vi "YMD.vi"() -> (0 "DD":string, 1 "MM":string, 2 "YYYY":string)   [LabVIEW 2013]
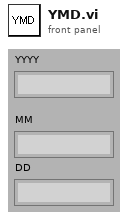
[diagram p1: front panel]
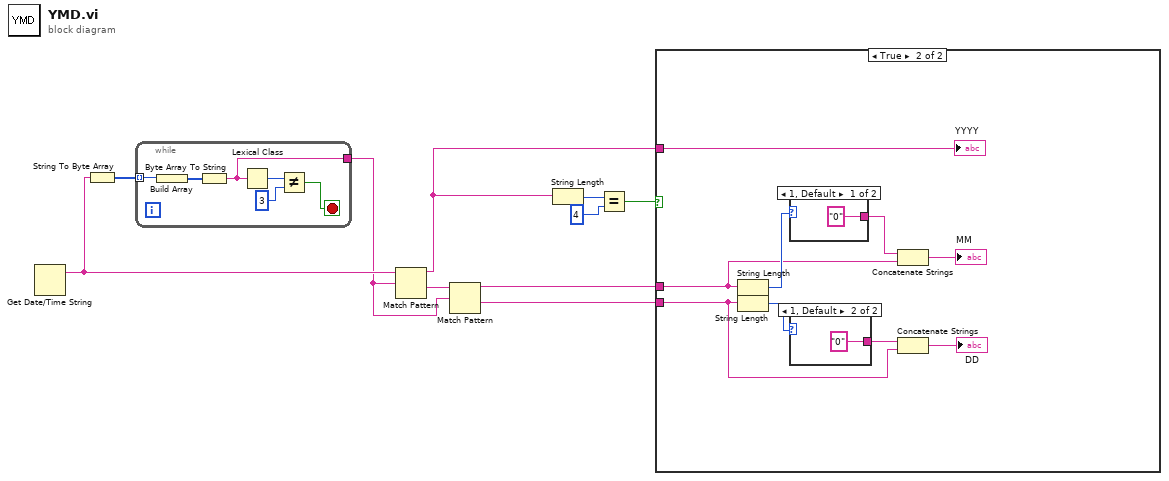
[diagram p0: block diagram]
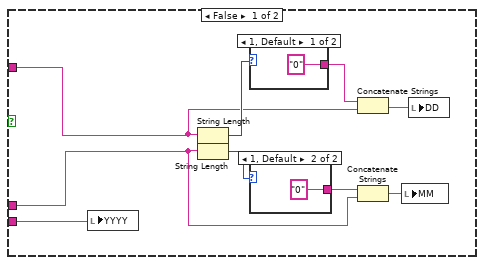
[diagram p2: hidden frame]
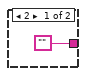
[diagram p3: hidden frame]
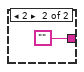
[diagram p4: hidden frame]
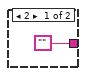
[diagram p5: hidden frame]
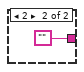
[diagram p6: hidden frame]
diagram:
  n1 = Get Date/Time String() -> (date string=w7:string)  [unwired: 4 out]
  n2 = String To Byte Array(string=w7) -> (unsigned byte array=w6:u8[])
  n3 = while {
    tunnel: w6 -> [w16] mode=indexing
    tunnel: [w11] -> w5
    stop <- w12 stop-if-true
    n4 = Build Array(w16) -> (w15:u8[])
    n5 = Byte Array To String(unsigned byte array=w15) -> (string=w11:string)
    n6 = Lexical Class(1:w11) -> (0:w14:i16)
    n7 = Not Equal?(x=w14, y=3) -> (x != y?=w12:bool)
  }
  n8 = Match Pattern(string=w7, regular expression=w5) -> (before substring=w4:string, after substring=w8:string)  [unwired: 3 out]
  n9 = Match Pattern(string=w8, regular expression=w5) -> (before substring=w9:string, after substring=w10:string)  [unwired: 3 out]
  n10 = String Length(string=w4) -> (length=w3:i32)
  n11 = Equal?(x=w3, y=4) -> (x = y?=w1:bool)
  n12 = case shown="True" w1 {
    tunnel: w10 -> [w19 w35]
    tunnel: w9 -> [w20 w33]
    tunnel: w4 -> [w21 w30]
    frame False {
      n13 = local write "YYYY"(w19) -> ()
      n14 = String Length(string=w21) -> (length=w25:i32)
      n15 = String Length(string=w20) -> (length=w24:i32)
      n16 = case shown="1, Default" w25 {
        tunnel: ["0" ""] -> w22
        frame 1, Default {
        }
        frame 2 {
        }
      }
      n17 = case shown="1, Default" w24 {
        tunnel: ["" "0"] -> w23
        frame 2 {
        }
        frame 1, Default {
        }
      }
      n18 = Concatenate Strings(w22, w21) -> (w17:string)
      n19 = Concatenate Strings(w23, w20) -> (w18:string)
      n20 = local write "MM"(w18) -> ()
      n21 = local write "DD"(w17) -> ()
    }
    frame True {
      n22 = String Length(string=w33) -> (length=w38:i32)
      n23 = String Length(string=w35) -> (length=w37:i32)
      n24 = case shown="1, Default" w38 {
        tunnel: ["0" ""] -> w34
        frame 1, Default {
        }
        frame 2 {
        }
      }
      n25 = case shown="1, Default" w37 {
        tunnel: ["" "0"] -> w36
        frame 2 {
        }
        frame 1, Default {
        }
      }
      n26 = Concatenate Strings(w34, w33) -> (→"MM":string)
      n27 = Concatenate Strings(w36, w35) -> (→"DD":string)
      "YYYY" <- w30
    }
  }
